vi "Ensure Discovery Service Started.vi"(8 "error in":errorcluster, 10 "cluster id":string, 11 "path":path) -> (0 "error out":errorcluster, 3 "key file path":path)   [LabVIEW 2020, in "Plug-In SDK Discovery V1 API.lvlib"]
uses:
  Plug-In SDK Discovery V1 API.lvlib
  <vilib>/ErrorRing/Error Ring.xnode
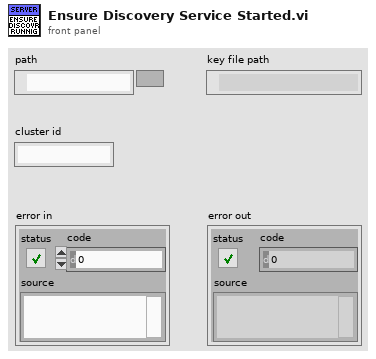
[diagram p1: front panel]
types:
  T1 = enum16{"open", "replace", "create", "open or create", "replace or create", "replace or create with confirmation"}
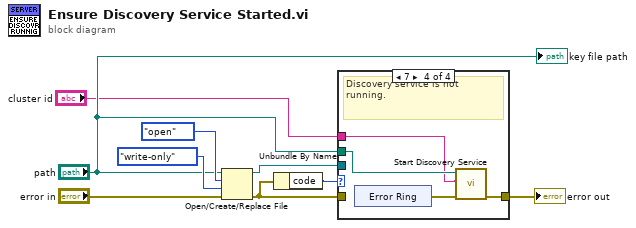
[diagram p0: block diagram]
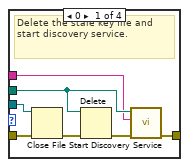
[diagram p2: hidden frame]
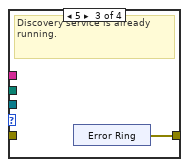
[diagram p4: hidden frame]
diagram:
  n1 = Open/Create/Replace File(file path (use dialog)="path", error in="error in", operation (0:open)=T1."open", access (0:read/write)=enum16{"read/write", "read-only", "write-only"}."write-only") -> (refnum out=w6:refnum<file>, error out=w4:errorcluster)  [unwired: 2 in, 1 out]
  n2 = Unbundle By Name(w4) -> ("code"=w5:i32)
  n3 = case shown="7" w5 {
    tunnel: w6 -> [w16 _ _ _]
    tunnel: [w13 w17 w18 w23] -> w3
    tunnel: w4 -> [w11 w17 _ _]
    tunnel: "path" -> [w12 _ _ w22]
    tunnel: "cluster id" -> [w10 _ _ w20]
    frame 0 {
      # "Delete the stale key file and start discovery service."
      n4 = Close File(refnum=w16, error in=w11) -> (error out=w15:errorcluster)  [unwired: 1 out]
      n5 = Delete(path (use dialog)=w12, error in=w15) -> (error out=w14:errorcluster)  [unwired: 3 in, 2 out]
      n6 = call "Start Discovery Service.vi"("error in"=w14, "cluster id"=w10, "key file path"=w12) -> ("error out"=w13:errorcluster)  [unwired: 8 in]
    }
    frame 1, Default {
      # "Error occurred in any of the previous node."
    }
    frame 5 {
      # "Discovery service is already running."
      n7 = xnode "Error Ring"() -> ("error out"=w18:errorcluster)
    }
    frame 7 {
      # "Discovery service is not running."
      n8 = xnode "Error Ring"() -> ("error out"=w21:errorcluster)
      n9 = call "Start Discovery Service.vi"("error in"=w21, "cluster id"=w20, "key file path"=w22) -> ("error out"=w23:errorcluster)  [unwired: 8 in]
    }
  }
  "error out" <- w3
  "key file path" <- "path"
